vi "Update Model Info.vi"(8 "error in (no error)":errorcluster, 11 "Loop Data":T1) -> (0 "error out":errorcluster)   [LabVIEW 2016, in "System Mapping Tool.lvlib"]
uses:
  System Mapping Tool.lvlib
  TypeDefs/Model Analysis Data.ctl
  TypeDefs/Model Analysis UI Refs.ctl
  NationalInstruments.VeriStand.SystemStorageUI
  NationalInstruments.VeriStand.SystemDefinitionAPI
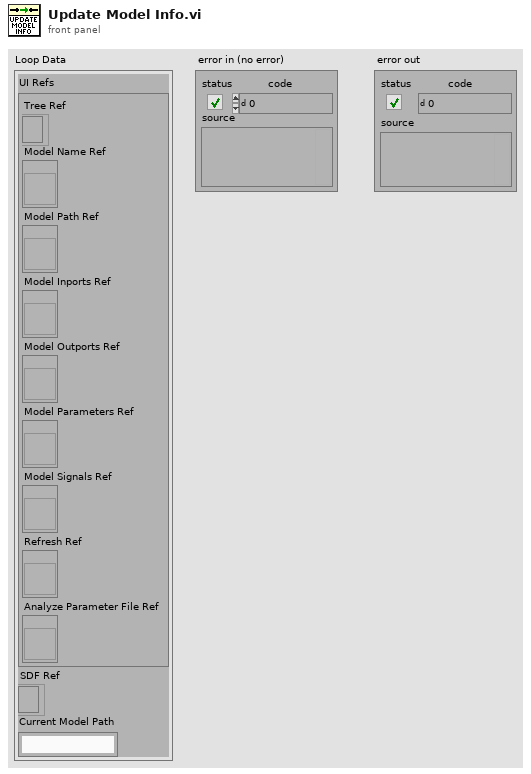
[diagram p1: front panel]
types:
  T1 = typedef "System Mapping Tool.lvlib/Model Analysis Data.ctl" = cluster{"UI Refs":T2, "SDF Ref":refnum<k24>, "Current Model Path":string}
  T2 = typedef "System Mapping Tool.lvlib/Model Analysis UI Refs.ctl" = cluster{"Tree Ref":refnum<k24>, "Model Name Ref":refnum<vi>, "Model Path Ref":refnum<vi>, "Model Inports Ref":refnum<vi>, "Model Outports Ref":refnum<vi>, "Model Parameters Ref":refnum<vi>, "Model Signals Ref":refnum<vi>, "Refresh Ref":refnum<vi>, "Analyze Parameter File Ref":refnum<vi>}
  T3 = enum8{"Enabled", "Disabled", "Disabled and Grayed Out"}
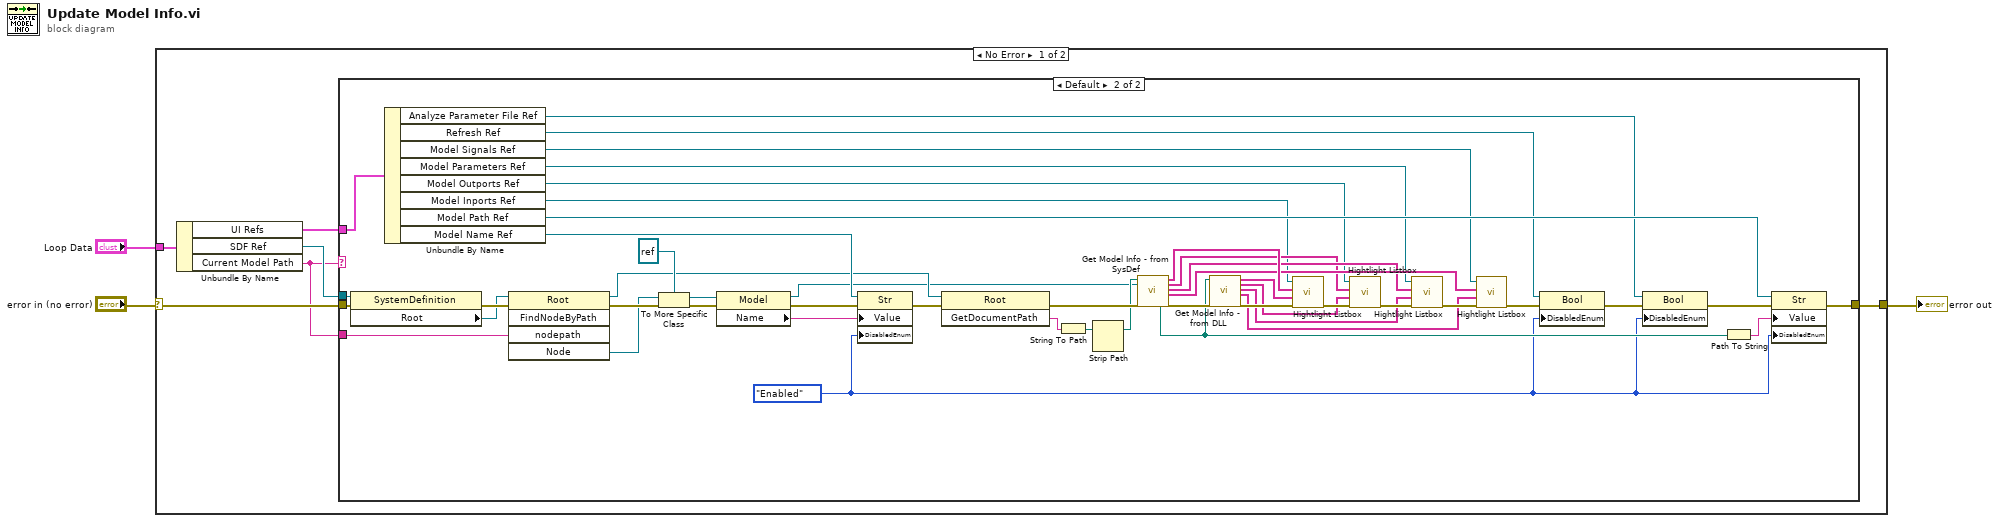
[diagram p0: block diagram]
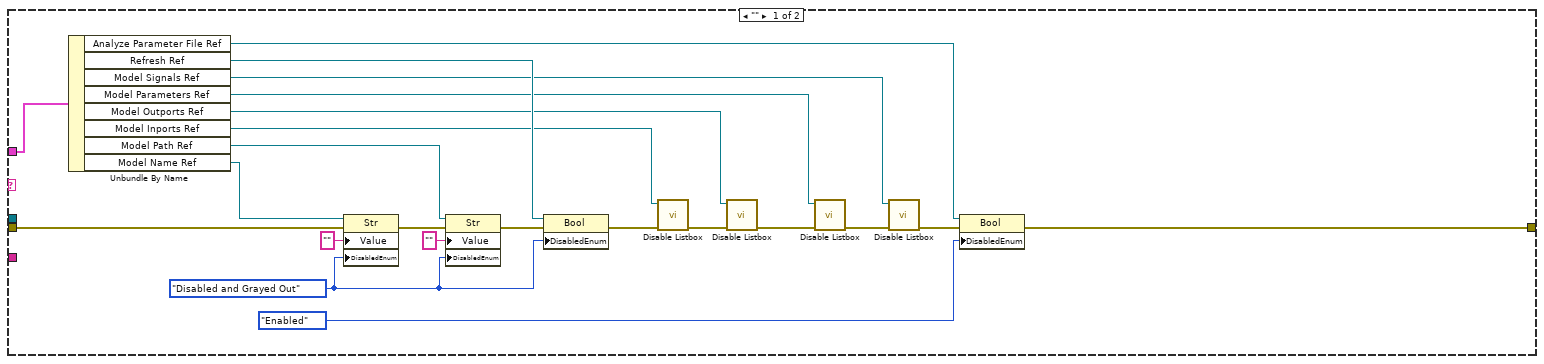
[diagram p2: hidden frame]
diagram:
  n1 = case shown="No Error" "error in (no error)" {
    selector: "error in (no error)" -> [w8 w80]
    tunnel: [w5 w80] -> w2
    tunnel: "Loop Data" -> [w9 _]
    frame No Error {
      n2 = Unbundle By Name(w9) -> ("UI Refs"=w4:T2, "SDF Ref"=w7:refnum<k24>, "Current Model Path"=w6:string)
      n3 = case shown="Default" w6 {
        tunnel: w8 -> [w30 w79]
        tunnel: w7 -> [_ w65]
        tunnel: w6 -> [_ w77]
        tunnel: [w11 w38] -> w5
        tunnel: w4 -> [w29 w71]
        frame "" {
          w13 = T3."Disabled and Grayed Out" ("Disabled")
          n4 = Unbundle By Name(w29) -> ("Analyze Parameter File Ref"=w12:refnum<vi>, "Refresh Ref"=w24:refnum<vi>, "Model Signals Ref"=w18:refnum<vi>, "Model Parameters Ref"=w17:refnum<vi>, "Model Outports Ref"=w16:refnum<vi>, "Model Inports Ref"=w15:refnum<vi>, "Model Path Ref"=w25:refnum<vi>, "Model Name Ref"=w28:refnum<vi>)
          n5 = property class="Str"(reference=w28, error in=w30, "Value"="", "DisabledEnum"=w13) -> (error out=w31:errorcluster)  [unwired: 1 out]
          n6 = property class="Str"(reference=w25, error in=w31, "Value"="", "DisabledEnum"=w13) -> (error out=w23:errorcluster)  [unwired: 1 out]
          n7 = property class="Bool"(reference=w24, error in=w23, "DisabledEnum"=w13) -> (error out=w22:errorcluster)  [unwired: 1 out]
          n8 = call "Disable Listbox.vi"("error in (no error)"=w22, "Listbox Ref"=w15) -> ("error out"=w21:errorcluster)  [unwired: 9 in]
          n9 = call "Disable Listbox.vi"("error in (no error)"=w21, "Listbox Ref"=w16) -> ("error out"=w20:errorcluster)  [unwired: 9 in]
          n10 = call "Disable Listbox.vi"("error in (no error)"=w20, "Listbox Ref"=w17) -> ("error out"=w19:errorcluster)  [unwired: 9 in]
          n11 = call "Disable Listbox.vi"("error in (no error)"=w19, "Listbox Ref"=w18) -> ("error out"=w14:errorcluster)  [unwired: 9 in]
          n12 = property class="Bool"(reference=w12, error in=w14, "DisabledEnum"=T3."Enabled" ("Disabled")) -> (error out=w11:errorcluster)  [unwired: 1 out]
        }
        frame Default {
          w33 = T3."Enabled" ("Disabled")
          n13 = property class="SystemDefinition"(reference=w65, error in=w79) -> (error out=w78:errorcluster, "Root"=w64:refnum<k24>)  [unwired: 1 out]
          n14 = Unbundle By Name(w71) -> ("Analyze Parameter File Ref"=w32:refnum<vi>, "Refresh Ref"=w67:refnum<vi>, "Model Signals Ref"=w41:refnum<vi>, "Model Parameters Ref"=w42:refnum<vi>, "Model Outports Ref"=w43:refnum<vi>, "Model Inports Ref"=w44:refnum<vi>, "Model Path Ref"=w68:refnum<vi>, "Model Name Ref"=w70:refnum<vi>)
          n15 = invoke class="Root" method="FindNodeByPath"(reference=w64, error in=w78, "nodepath"=w77) -> (reference out=w61:refnum<k24>, error out=w76:errorcluster, "Node"=w75:refnum<k24>)  [unwired: 2 in, 2 out]
          n16 = To More Specific Class(target class=refnum<k24> refnum (".NET object"), reference=w75, error in=w76) -> (specific class reference=w74:refnum<k24>, error out=w66:errorcluster)
          n17 = property class="Model"(reference=w74, error in=w66) -> (reference out=w58:refnum<k24>, error out=w72:errorcluster, "Name"=w69:string)
          n18 = property class="Str"(reference=w70, error in=w72, "Value"=w69, "DisabledEnum"=w33) -> (error out=w39:errorcluster)  [unwired: 1 out]
          n19 = invoke class="Root" method="GetDocumentPath"(reference=w61, error in=w39) -> (error out=w60:errorcluster, "GetDocumentPath"=w62:string)  [unwired: 1 in, 1 out]
          n20 = String To Path(string=w62) -> (path=w63:path)
          n21 = Strip Path(path=w63) -> (stripped path=w59:path)  [unwired: 1 out]
          n22 = call "Get Model Info - from SysDef.vi"("System Definition Filepath (.nivssdf)"=w59, "Model Ref"=w58, "Error (in)"=w60) -> ("Model Path"=w37:path, "SysDef Inports"=w52:string[], "SysDef Outports"=w45:string[], "SysDef Parameters"=w48:string[], "SysDef Signals"=w49:string[], "Error (out)"=w57:errorcluster)  [unwired: 10 in, 1 out]
          n23 = call "Get Model Info - from DLL.vi"("Model Filepath"=w37, "Error (in)"=w57) -> ("DLL Inports"=w51:string[], "DLL Outports"=w46:string[], "DLL Parameters"=w47:string[], "DLL Signals"=w50:string[], "Error (out)"=w56:errorcluster)  [unwired: 13 in]
          n24 = call "Hightlight Listbox.vi"("error in (no error)"=w56, "From DLL"=w51, "From SDF"=w52, "Listbox Ref"=w44) -> ("error out"=w55:errorcluster)  [unwired: 7 in]
          n25 = call "Hightlight Listbox.vi"("error in (no error)"=w55, "From DLL"=w46, "From SDF"=w45, "Listbox Ref"=w43) -> ("error out"=w54:errorcluster)  [unwired: 7 in]
          n26 = call "Hightlight Listbox.vi"("error in (no error)"=w54, "From DLL"=w47, "From SDF"=w48, "Listbox Ref"=w42) -> ("error out"=w53:errorcluster)  [unwired: 7 in]
          n27 = call "Hightlight Listbox.vi"("error in (no error)"=w53, "From DLL"=w50, "From SDF"=w49, "Listbox Ref"=w41) -> ("error out"=w40:errorcluster)  [unwired: 7 in]
          n28 = property class="Bool"(reference=w67, error in=w40, "DisabledEnum"=w33) -> (error out=w35:errorcluster)  [unwired: 1 out]
          n29 = property class="Bool"(reference=w32, error in=w35, "DisabledEnum"=w33) -> (error out=w34:errorcluster)  [unwired: 1 out]
          n30 = Path To String(path=w37) -> (string=w36:string)
          n31 = property class="Str"(reference=w68, error in=w34, "Value"=w36, "DisabledEnum"=w33) -> (error out=w38:errorcluster)  [unwired: 1 out]
        }
      }
    }
    frame Error {
    }
  }
  "error out" <- w2
